vi "Calibrate Gripper.vi"(8 "error in (no error)":errorcluster, 11 "KUKA youBot gripper in":refnum<class "NI_Robotics_KUKA youBot Gripper_EtherCAT.lvclass">) -> (0 "error out":errorcluster, 3 "KUKA youBot gripper out":refnum<class "NI_Robotics_KUKA youBot Gripper_EtherCAT.lvclass">)   [LabVIEW 2017, in "NI_Robotics_KUKA youBot Host.lvlib" / "NI_Robotics_KUKA youBot Gripper_EtherCAT.lvclass"]
uses:
  <vilib>/robotics/KUKA youBot/Basic Device/Gripper EtherCAT/NI_Robotics_KUKA youBot Gripper_EtherCAT.lvclass
  <vilib>/robotics/KUKA youBot/Motor/Gripper Motor/NI_Robotics_KUKA youBot Gripper Motor.lvclass
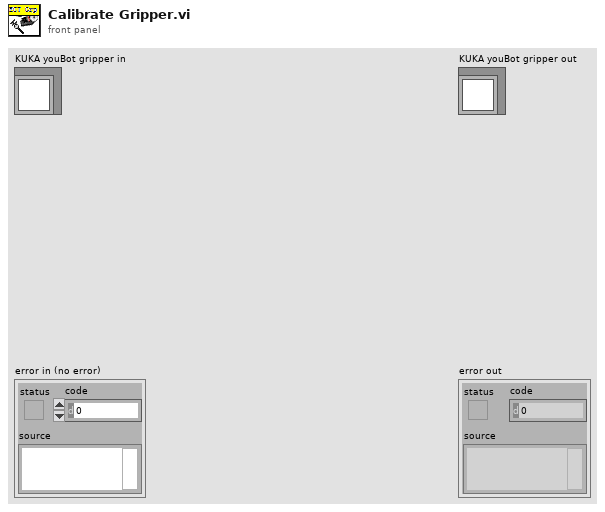
[diagram p1: front panel]
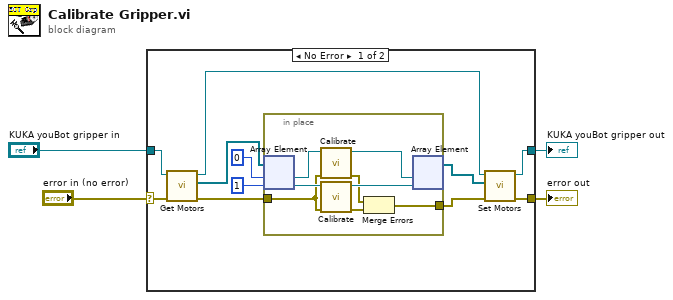
[diagram p0: block diagram]
diagram:
  n1 = case shown="No Error" "error in (no error)" {
    selector: "error in (no error)" -> [w14 w25]
    tunnel: "KUKA youBot gripper in" -> [w15 w24]
    tunnel: [w12 w24] -> w2
    tunnel: [w11 w25] -> w1
    frame No Error {
      n2 = call-dynamic "Get Motors.vi"("error in (no error)"=w14, "KUKA youBot gripper in"=w15) -> ("error out"=w9:errorcluster, "motors"=w10:refnum<class "NI_Robotics_KUKA youBot Gripper Motor.lvclass">[], "KUKA youBot gripper out"=w13:refnum<class "NI_Robotics_KUKA youBot Gripper_EtherCAT.lvclass">)  [unwired: 7 in]
      n3 = in-place {
        in-place-border: w9 -> [w19]
        in-place-border: [w16] -> w7
        n4 = in-place-array #1(w10, 0, 1) -> (w23:refnum<class "NI_Robotics_KUKA youBot Gripper Motor.lvclass">, w21:refnum<class "NI_Robotics_KUKA youBot Gripper Motor.lvclass">)
        n5 = call-dynamic "Calibrate.vi"("error in (no error)"=w19, "KUKA youBot gripper motor in"=w23) -> ("error out"=w18:errorcluster, "KUKA youBot gripper motor out"=w22:refnum<class "NI_Robotics_KUKA youBot Gripper Motor.lvclass">)  [unwired: 8 in]
        n6 = call-dynamic "Calibrate.vi"("error in (no error)"=w19, "KUKA youBot gripper motor in"=w21) -> ("error out"=w17:errorcluster, "KUKA youBot gripper motor out"=w20:refnum<class "NI_Robotics_KUKA youBot Gripper Motor.lvclass">)  [unwired: 8 in]
        n7 = Merge Errors(w18, w17) -> (w16:errorcluster)
        n8 = in-place-array #1(w22, w20) -> (w8:refnum<class "NI_Robotics_KUKA youBot Gripper Motor.lvclass">[])  [unwired: 2 out]
      }
      n9 = call-dynamic "Set Motors.vi"("error in (no error)"=w7, "motors"=w8, "KUKA youBot gripper in"=w13) -> ("error out"=w11:errorcluster, "KUKA youBot gripper out"=w12:refnum<class "NI_Robotics_KUKA youBot Gripper_EtherCAT.lvclass">)  [unwired: 7 in]
    }
    frame Error {
    }
  }
  "error out" <- w1
  "KUKA youBot gripper out" <- w2
